vi "Untitled 3 (SubVI).vi"(11 "Numeric":i32) -> (3 "msg out":string)   [LabVIEW 2016]
uses:
  builds/UnicornMain/UnicornRIO1/ROS for LabVIEW/home/lvuser/natinst/bin/user.lib/ROS for LabVIEW Software/ROS/MessageBuilding/std_msgs/subs/i32Scalar.vi
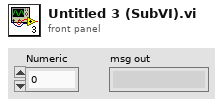
[diagram p1: front panel]
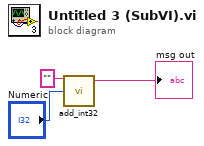
[diagram p0: block diagram]
diagram:
  n1 = call-poly "add_int32.vi"("Numeric"="Numeric", "msg in"="") -> ("msg out"=→"msg out":string)  [unwired: 3 in]
